vi "RefnameToString.vi"(1 "Enum":T1) -> (0 "Refname":string)   [LabVIEW 2012]
uses:
  RefnameEnum.ctl
panel:
  in  "RefnameArray":string[](array[string])=["FireLauncher", "Climber", "Shield", "TankDrive", "DriveEncoderL", "DriveEncoderR", "LauncherMotorRPM", "LauncherEncoderAnalog", "LauncherEncoderRPM", "ShooterLS", "DriveAlignLSLeft", "DriveAlignLSRight", "ClimbingLS", "LauncherEncoderAngle", "LauncherMotorAngle", "Gamepad1", "Gamepad2", "Compressor", "ClimbWeightSol3", "ClimbWeightSol4"]
  # "SET CHANGED VALUES\nAS DEFAULTS!!!"
  # "SET CHANGED VALUES\nAS DEFAULTS!!!"
  # "SET CHANGED VALUES\nAS DEFAULTS!!!"
  # "SET CHANGED VALUES\nAS DEFAULTS!!!"
  # "SET CHANGED VALUES\nAS DEFAULTS!!!"
  # "SET CHANGED VALUES\nAS DEFAULTS!!!"
  # "SET CHANGED VALUES\nAS DEFAULTS!!!"
  # "SET CHANGED VALUES\nAS DEFAULTS!!!"
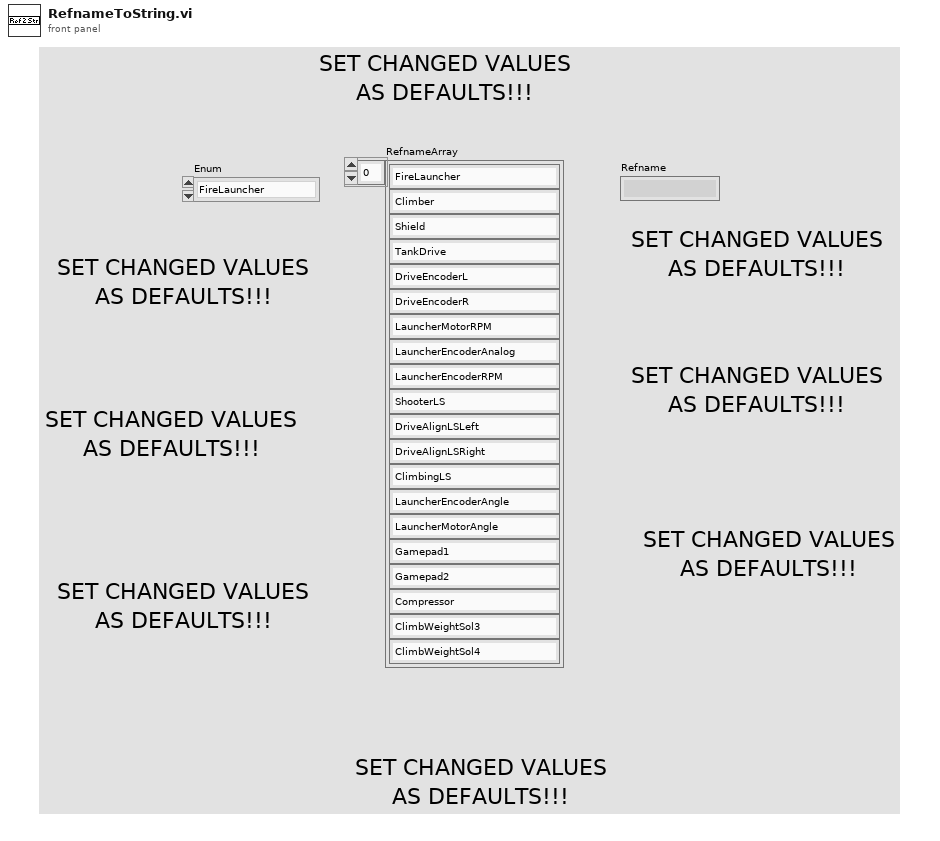
[diagram p1: front panel]
types:
  T1 = typedef "RefnameEnum.ctl" = enum16{"FireLauncher", "Climber", "Shield", "TankDrive", "DriveEncoderL", "DriveEncoderR", "LauncherMotorRPM", "LauncherEncoderAnalog", "LauncherEncoderRPM", "ShooterLS", "DriveAlignLSLeft", "DriveAlignLSRight", "ClimbingLS", "LauncherEncoderAngle", "LauncherMotorAngle", "Gamepad1", "Gamepad2", "Compressor", "ClimbWeightSol3", "ClimbWeightSol4"}
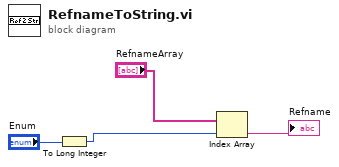
[diagram p0: block diagram]
diagram:
  n1 = To Long Integer(number="Enum") -> (32bit integer=w1:i32)
  n2 = Index Array(array="RefnameArray", index=w1) -> (element=→"Refname":string)
